vi "Simple Encoder Test 1.vi"() -> ()   [LabVIEW 2014]
uses:
  <vilib>/LabVIEW Universal Transcriptor/LabVIEW to Arduino Transcriptor/Transcriptors/System API/Serial println string.vi
  Encoder.lvclass
panel:
  out "Error Out":errorcluster
  in  "error in":errorcluster
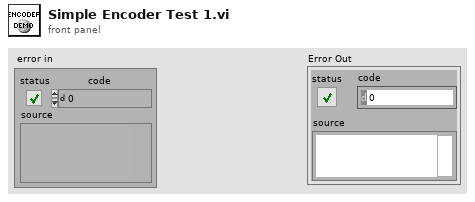
[diagram p1: front panel]
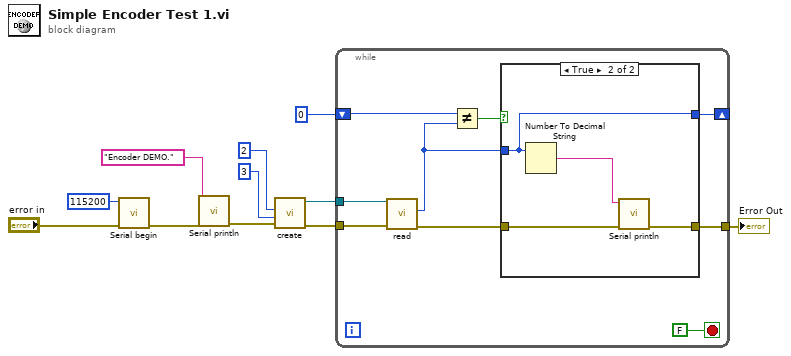
[diagram p0: block diagram]
diagram:
  n1 = call <vilib>:"Serial begin.vi"("Error In"="error in", "speed (Bd)"=115200) -> ("Error Out"=w6:errorcluster)  [unwired: 9 in]
  n2 = call-poly <vilib>:"Serial println.vi"("Error In"=w6, "string in"="Encoder DEMO.") -> ("Error Out"=w5:errorcluster)  [unwired: 9 in]
  n3 = call "create.vi"("error in"=w5, "pin2"=u8 3 ("pin1"), "pin1"=u8 2) -> ("error out"=w10:errorcluster, "Encoder in"=w9:refnum<class "Encoder.lvclass">)  [unwired: 7 in]
  n4 = while {
    tunnel: w10 -> [w19]
    tunnel: w9 -> [w18]
    tunnel: [w13] -> w3
    shift-right: [w12] -> _
    shift-left: 0 -> [w17]
    stop <- FALSE stop-if-true
    n5 = call "read.vi"("error in (no error)"=w19, "Encoder in"=w18) -> ("error out"=w15:errorcluster, "value"=w14:i32)  [unwired: 7 in]
    n6 = Not Equal?(x=w17, y=w14) -> (x != y?=w16:bool)
    n7 = case shown="True" w16 {
      tunnel: w15 -> [w22 w25]
      tunnel: w14 -> [w21 w23]
      tunnel: [w22 w24] -> w13
      tunnel: [w21 w23] -> w12
      frame False {
      }
      frame True {
        n8 = Number To Decimal String(number=w23) -> (decimal integer string=w26:string)  [unwired: 1 in]
        n9 = call-poly <vilib>:"Serial println.vi"("Error In"=w25, "string in"=w26) -> ("Error Out"=w24:errorcluster)  [unwired: 9 in]
      }
    }
  }
  "Error Out" <- w3
